vi "AO_6711_Run_Async.vi"(8 "error in (no error)":errorcluster, 11 "Instrument handle in":refnum<k21>) -> (0 "error out":errorcluster)   [LabVIEW 2020]
doc: "This VI runs asynchronously. It starts a waveform generation in response to one or many triggers, and waits until the end of the generation before to stop."
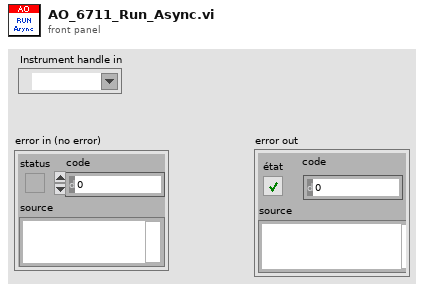
[diagram p1: front panel]
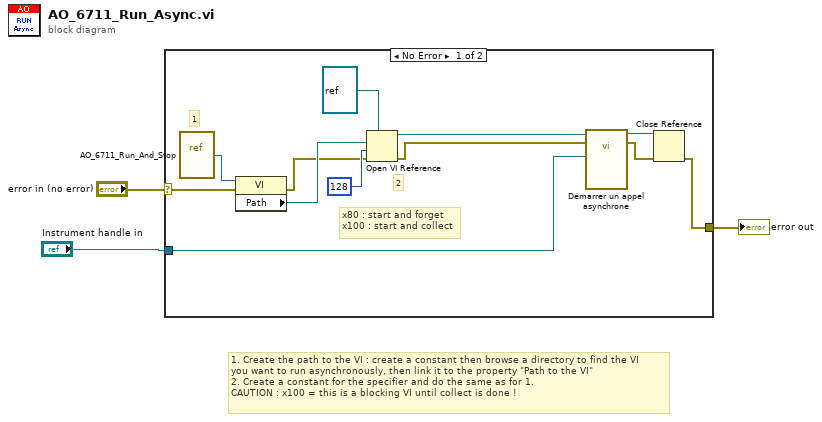
[diagram p0: block diagram]
diagram:
  # "1. Create the path to the VI : create a constant then browse a directory to find the VI\nyou want to run asynchronously, then link it to the property \"Path to the VI\"\n2. Create a constant for the specifier and do the same as for 1.\nCAUTION : x100 = this is a blocking VI until collect is done !"
  n1 = case shown="No Error" "error in (no error)" {
    selector: "error in (no error)" -> [w13 w16]
    tunnel: [w4 w16] -> w2
    tunnel: "Instrument handle in" -> [w7 _]
    frame No Error {
      # "1"
      # "2"
      # "x80 : start and forget\nx100 : start and collect"
      n2 = vi-ref "AO_6711_Run_And_Stop.vi"() -> (w10:refnum<vi>)
      n3 = property class="VI"(reference=w10, error in=w13) -> (error out=w12:errorcluster, "Path"=w14:path)  [unwired: 1 out]
      n4 = Open VI Reference(type specifier VI Refnum (for type only)=refnum<vi> refnum ("spécificateur de type du refnum de VI (pour type seulement)"), vi path=w14, options=128, error in (no error)=w12) -> (vi reference=w8:refnum<vi>, error out=w11:errorcluster)  [unwired: 2 in]
      n5 = call-by-ref "Démarrer un appel asynchrone"(reference=w8, error in=w11, "Instrument handle in"=w7) -> (reference out=w6:refnum<vi>, error out=w5:errorcluster)  [unwired: 10 in, 1 out]
      n6 = Close Reference(reference=w6, error in (no error)=w5) -> (error out=w4:errorcluster)
    }
    frame Error {
    }
  }
  "error out" <- w2
